vi "Read Data Bits.vi"(8 "error in (no error)":errorcluster, 11 "serial data unit in":refnum<class "Serial Data Unit.lvclass">) -> (0 "error out":errorcluster, 2 "data bits":u16=8, 3 "serial data unit out":refnum<class "Serial Data Unit.lvclass">)   [LabVIEW 2020, in "SubVIs.lvlib" / "Serial Data Unit.lvclass"]
doc: "Acts as a constant, and provides a way for the serial slave to properly configure the serial interface."
uses:
  <vilib>/Modbus/subvis/Transmission Data Unit (ADU)/Serial Data Unit/Serial Data Unit.lvclass
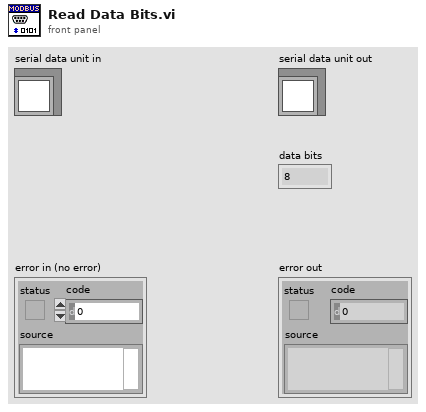
[diagram p1: front panel]
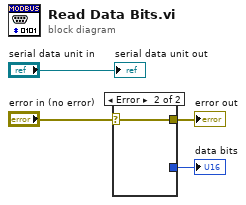
[diagram p0: block diagram]
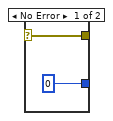
[diagram p2: hidden frame]
diagram:
  n1 = case shown="Error" "error in (no error)" {
    selector: "error in (no error)" -> [w5 w7]
    tunnel: [u16 0 ("data bits") _] -> w3
    tunnel: [w5 w7] -> w1
    frame No Error {
    }
    frame Error {
    }
  }
  "error out" <- w1
  "data bits" <- w3
  "serial data unit out" <- "serial data unit in"
